vi "save_image.vi"(10 "picture":picture, 11 "path to JPEG file":path) -> ()   [LabVIEW 2021]
uses:
  <vilib>/picture/picture.llb/imagedata.ctl
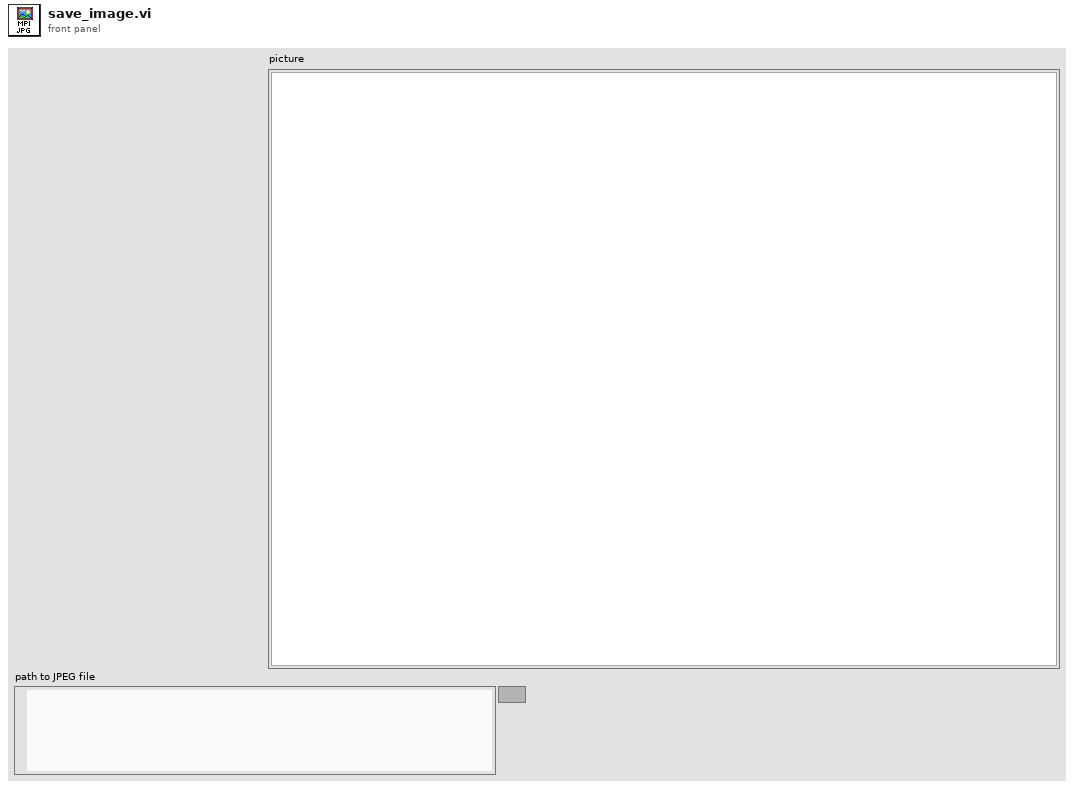
[diagram p1: front panel]
types:
  T1 = typedef "imagedata.ctl" = cluster{"image type":i32, "image depth":i32, "image":u8[], "mask":u8[], "colors":u32[], "Rectangle":cluster{"left":i16, "top":i16, "right":i16, "bottom":i16}}
  T2 = cluster{"left":i16, "top":i16, "right":i16, "bottom":i16}
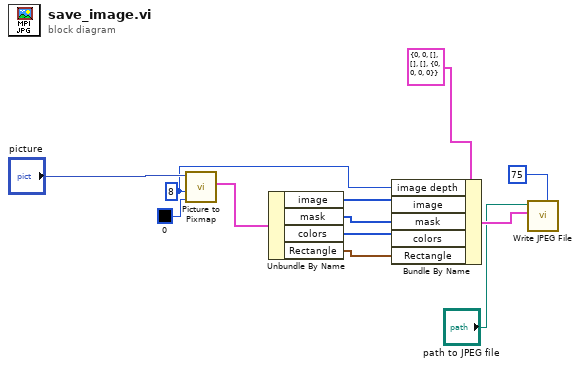
[diagram p0: block diagram]
diagram:
  w3 = 8 ("depth")
  n1 = call <vilib>:"Picture to Pixmap.vi"("Background Color"=u32 0, "depth"=w3, "picture"="picture") -> ("image data"=w10:T1)  [unwired: 7 in, 1 out]
  n2 = Unbundle By Name(w10) -> ("image"=w8:u8[], "mask"=w7:u8[], "colors"=w6:u32[], "Rectangle"=w5:T2)
  n3 = Bundle By Name(cluster=T1 {"image type"=0, "image depth"=0, "image"=[], "mask"=[], "colors"=[], "Rectangle"={"left"=0, "top"=0, "right"=0, "bottom"=0}} ("image data"), "image depth"=w3, "image"=w8, "mask"=w7, "colors"=w6, "Rectangle"=w5) -> (w4:T1)
  n4 = call <vilib>:"Write JPEG File.vi"("quality (80)"=75, "image data"=w4, "path to JPEG file"="path to JPEG file") -> ()  [unwired: 7 in, 2 out]
